vi "Configure Pressure Lookup.vi"(8 "error in (no error)":errorcluster, 11 "APG in":refnum<class "APG.lvclass">) -> (0 "error out":errorcluster, 3 "APG out":refnum<class "APG.lvclass">)   [LabVIEW 2021, in "APG.lvclass"]
uses:
  APG.lvclass
  APG.lvclass/APG.ctl
  <vilib>/Utility/file.llb/Read Delimited Spreadsheet (DBL).vi
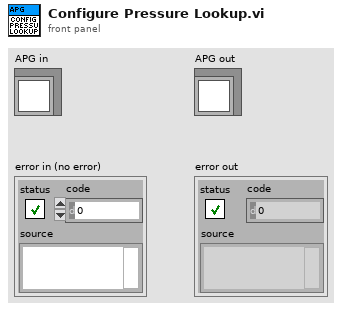
[diagram p1: front panel]
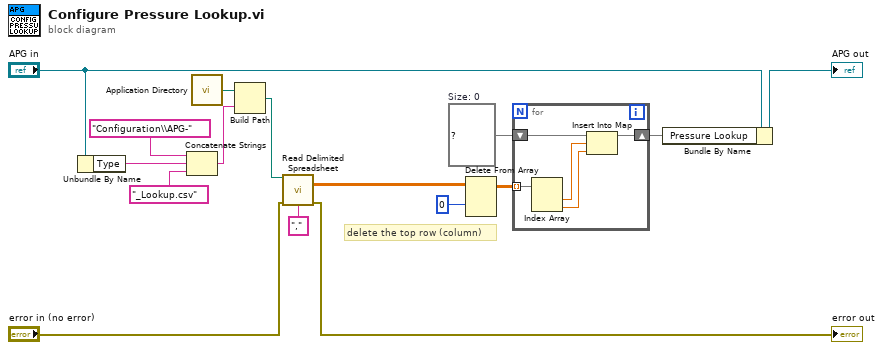
[diagram p0: block diagram]
diagram:
  w8 = map{dbl, dbl} {}  # Size: 0
  # "delete the top row (column)"
  n1 = Unbundle By Name("APG in") -> ("Type"=w2:string)
  n2 = Concatenate Strings("Configuration\\APG-", w2, "_Lookup.csv") -> (w1:string)
  n3 = call <vilib>:"Application Directory.vi"() -> ("Application Directory"=w14:path)
  n4 = Build Path(base path=w14, name or relative path=w1) -> (appended path=w15:path)
  n5 = call-poly <vilib>:"Read Delimited Spreadsheet.vi"("file path (dialog if empty)"=w15, "error in (no error)"="error in (no error)", "delimiter (\\t)"="," ("delimiter (\\t)")) -> ("all rows"=w12:dbl[][], "error out"=→"error out":errorcluster)  [unwired: 7 in, 4 out]
  n6 = Delete From Array(array=w12, index (row)=0) -> (array with subset deleted=w9:dbl[][])  [unwired: 2 in, 1 out]
  n7 = for {
    shift-right: [w20] -> w10
    shift-left: w8 -> [w21]
    tunnel: w9 -> [w19] mode=indexing
    n8 = Index Array(array=w19) -> (element #1=w18:dbl, element #2=w17:dbl)  [unwired: 2 in]
    n9 = Insert Into Map(map in=w21, key=w18, value=w17) -> (map out=w20:map{dbl, dbl})  [unwired: 2 out]
  }
  n10 = Bundle By Name(cluster="APG in", "Pressure Lookup"=w10) -> (→"APG out":refnum<class "APG.lvclass">)
